vi "SaveRingFiles.vi"(0 "h(r,t)":dbl[][](array[numeric]) format="%.2f", 2 "Path":path=path "E:/Test", 3 "Variables in":T1={"Number of rings"=1, "sound spd (cm/s)"=150000, "z span (cm)"=4.0, "z steps"=20, "number of y steps"=50, "y spacing (cm)"=0.01, "time step (s)"=1e-08, "z"=0.0, "y"=0.0, "ref delay"=0.0, "freq (MHz)"=4.71, "cycles"=300} {"freq (MHz)" format="%.2f"; "z span (cm)" format="%.2f"; "y" format="%.2f"; "ref delay" format="%.2f"; "y spacing (cm)" format="%.2f"; "z" format="%.2f"; "time step (s)" format="%.2e"}, 5 "Ring Number":i32) -> ()   [LabVIEW 2022 SP3]
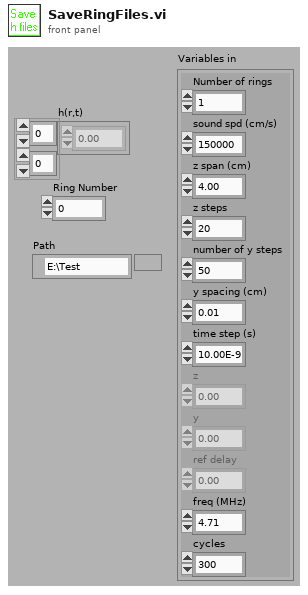
[diagram p1: front panel]
types:
  T1 = cluster{"Number of rings":i32, "sound spd (cm/s)":i32, "z span (cm)":dbl, "z steps":i32, "number of y steps":i32, "y spacing (cm)":dbl, "time step (s)":sgl, "z":dbl, "y":dbl, "ref delay":dbl, "freq (MHz)":dbl, "cycles":i32}
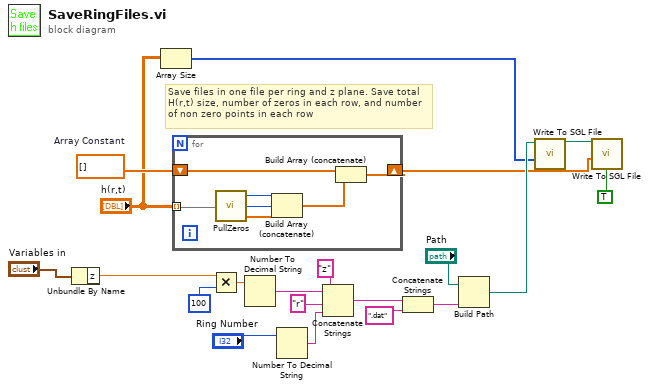
[diagram p0: block diagram]
diagram:
  w5 = sgl[] []  # Array Constant
  # "Save files in one file per ring and z plane. Save total H(r,t) size, number of zeros in each row, and number of non zero points in each row"
  n1 = Unbundle By Name("Variables in") -> ("z"=w20:dbl)
  n2 = Array Size(array="h(r,t)") -> (size(s)=w7:i32[])
  n3 = for {
    tunnel: "h(r,t)" -> [w25] mode=indexing
    shift-right: [w26] -> w3
    shift-left: w5 -> [w27]
    n4 = call "PullZeros.vi"("input"=w25) -> ("output"=w22:dbl[], "non zero points"=w23:i32, "pre-zeros"=w24:i32)  [unwired: 2 out]
    n5 = Build Array (concatenate)(w24, w23, w22) -> (w21:dbl[])
    n6 = Build Array (concatenate)(w27, w21) -> (w26:dbl[])
  }
  n7 = Multiply(x=w20, y=100) -> (x*y=w18:dbl)
  n8 = Number To Decimal String(number=w18) -> (decimal integer string=w17:string)  [unwired: 1 out]
  n9 = Number To Decimal String(number="Ring Number") -> (decimal integer string=w13:string)  [unwired: 1 out]
  n10 = Concatenate Strings("z", w17, "r", w13) -> (w12:string)
  n11 = Concatenate Strings(w12, ".dat") -> (w10:string)
  n12 = Build Path(base path="Path", name or relative path=w10) -> (appended path=w9:path)
  n13 = call <vilib>:"Write To SGL File.vi"("1D array"=w7, "file path (dialog if empty)"=w9) -> ("new file path (Not A Path if cancelled)"=w8:path)  [unwired: 2 in, 3 out]
  n14 = call <vilib>:"Write To SGL File.vi"("append to file? (new file:F)"=TRUE, "1D array"=w3, "file path (dialog if empty)"=w8) -> ()  [unwired: 1 in, 4 out]
